vi "Read loopCounter.vi"(8 "error in (no error)":errorcluster, 11 "ExampleTask_StopNotifier in":refnum<class "ExampleTask_BoolStopNotifier.lvclass">) -> (0 "error out":errorcluster, 2 "loopCounter":i32, 3 "ExampleTask_StopNotifier out":refnum<class "ExampleTask_BoolStopNotifier.lvclass">)   [LabVIEW 2023, in "ExampleTask_BoolStopNotifier.lvclass"]
uses:
  ExampleTask_BoolStopNotifier.lvclass
  ExampleTask_BoolStopNotifier.lvclass/ExampleTask_BoolStopNotifier.ctl
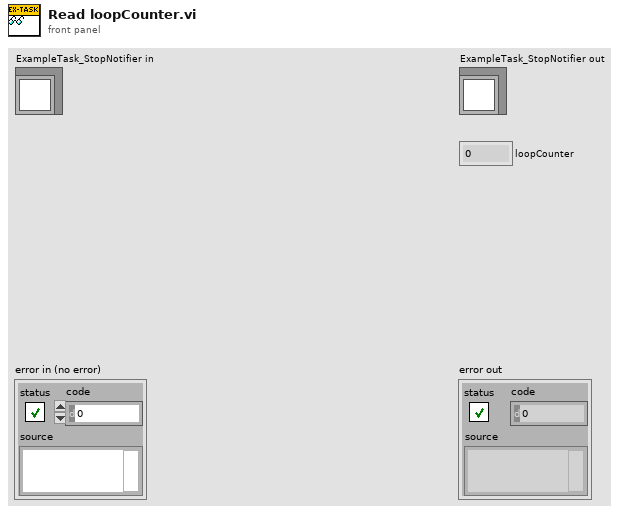
[diagram p1: front panel]
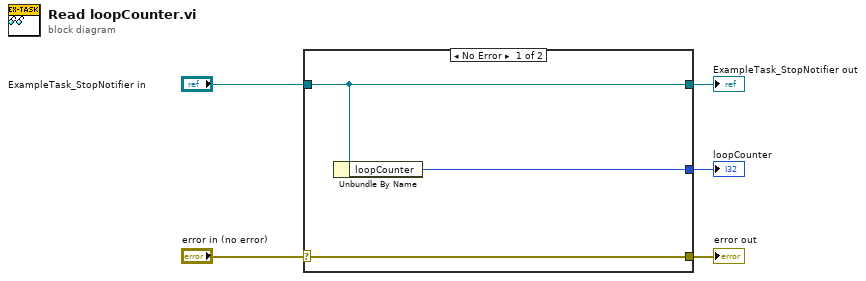
[diagram p0: block diagram]
diagram:
  n1 = case shown="No Error" "error in (no error)" {
    selector: "error in (no error)" -> [w8 w9]
    tunnel: [w8 w9] -> w4
    tunnel: [w7 w10] -> w2
    tunnel: "ExampleTask_StopNotifier in" -> [w7 w10]
    tunnel: [w6 _] -> w1
    frame No Error {
      n2 = Unbundle By Name(w7) -> ("loopCounter"=w6:i32)
    }
    frame Error {
    }
  }
  "error out" <- w4
  "ExampleTask_StopNotifier out" <- w2
  "loopCounter" <- w1
